vi "Configure S-parameter Table.vi"(6 "Operation (0: Active Existing Table)":i32(ring) items=["Active Existing Table"=0, "Define Frequency Array"=1, "Rename Existing Table"=3, "Clear Existing Table"=4], 7 "New Table Name (\"MyTable\")":string="MyTable", 8 "error in (no error)":errorcluster, 9 "Table Data":i32[](array[numeric]), 10 "S-parameter Table Name (\"DEFAULT\")":string="DEFAULT", 11 "VISA resource name":refnum<visa-resource-name>) -> (0 "error out":errorcluster, 3 "VISA resource name out":refnum<visa-resource-name>)   [LabVIEW 2018, in "Agilent U2000 Series.lvlib"]
doc: "Operates instrument for the S-parameter table functionality. Includes: Defines, Selects the S-parameter table to be used in the S-parameter correction, renames or clears specified S-parameter table. \n\nNote:\nThis VI is only applicable for U2040 X-Series."
uses:
  Agilent U2000 Series.lvlib
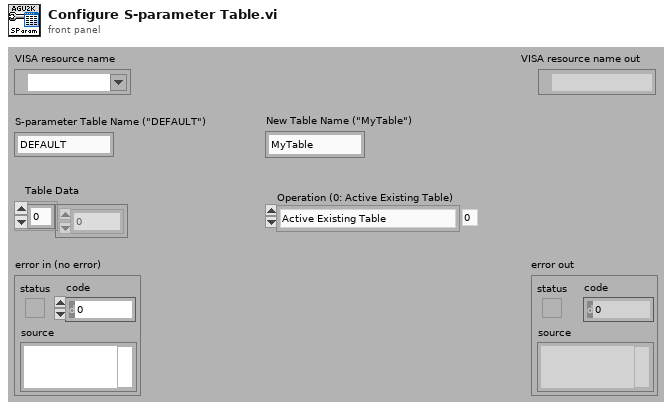
[diagram p1: front panel]
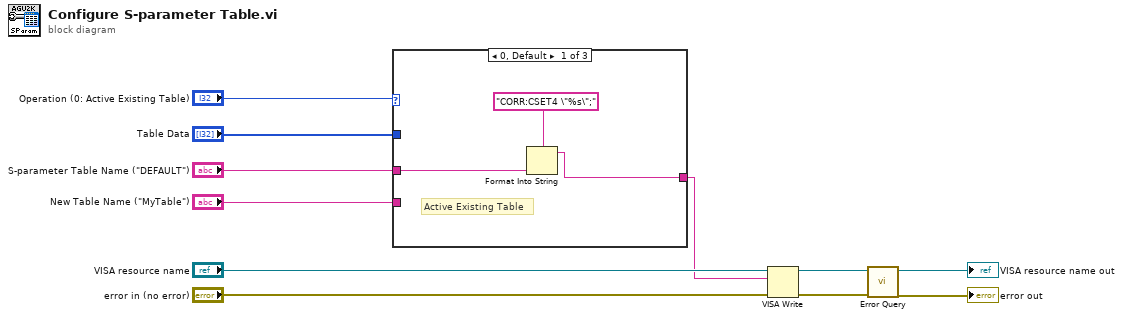
[diagram p0: block diagram]
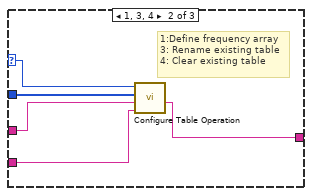
[diagram p2: hidden frame]
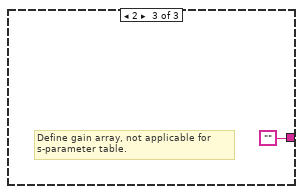
[diagram p3: hidden frame]
diagram:
  n1 = case shown="0, Default" "Operation (0: Active Existing Table)" {
    selector: "Operation (0: Active Existing Table)" -> [_ w19 _]
    tunnel: [w14 w15 ""] -> w2
    tunnel: "S-parameter Table Name (\"DEFAULT\")" -> [w12 w17 _]
    tunnel: "New Table Name (\"MyTable\")" -> [_ w16 _]
    tunnel: "Table Data" -> [_ w18 _]
    frame 0, Default {
      # "Active Existing Table"
      n2 = Format Into String(format string="CORR:CSET4 \"%s\";", w12) -> (resulting string=w14:string)  [unwired: 2 in, 1 out]
    }
    frame 1, 3, 4 {
      # "1:Define frequency array\n3: Rename existing table\n4: Clear existing table"
      n3 = call "Configure Table Operation.vi"("New Table Name (\"MyTable\")"=w16, "Table Name (\"DEFAULT\")"=w17, "Table Data"=w18, "Operation (1: Define Frequency Array)"=w19) -> ("ResultString"=w15:string)  [unwired: 7 in]
    }
    frame 2 {
      # "Define gain array, not applicable for s-parameter table."
    }
  }
  n4 = VISA Write(VISA resource name="VISA resource name", write buffer=w2, error in (no error)="error in (no error)") -> (VISA resource name out=w9:refnum<visa-resource-name>, error out=w8:errorcluster)  [unwired: 1 out]
  n5 = call "Error Query.vi"("error in (no error)"=w8, "VISA resource name"=w9) -> ("error out"=→"error out":errorcluster, "VISA resource name out"=→"VISA resource name out":refnum<visa-resource-name>)  [unwired: 6 in, 2 out]
